vi "Get Value.vi"(8 "error in (no error)":errorcluster, 11 "Node in":refnum<class "Node.lvclass">) -> (0 "error out":errorcluster, 2 "Value":string, 3 "Node out":refnum<class "Node.lvclass">)   [LabVIEW 2020, in "PicoG-ParserLexer.lvlib" / "Node.lvclass"]
uses:
  Node.lvclass
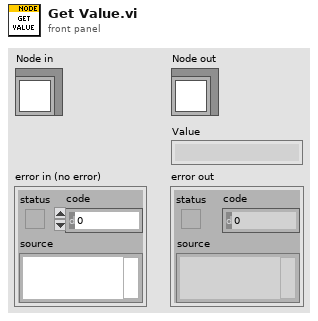
[diagram p1: front panel]
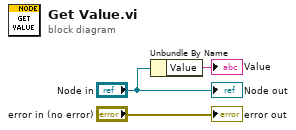
[diagram p0: block diagram]
diagram:
  n1 = Unbundle By Name("Node in") -> ("Value"=→"Value":string)
  "error out" <- "error in (no error)"
  "Node out" <- "Node in"
